vi "Handle Menu Selection.vi"(6 "Coords":T1, 8 "error in (no error)":errorcluster, 9 "Item Tag":string, 10 "Tree Refnum":refnum<vi>, 11 "Test Executive View in":refnum<class "Test Executive View.lvclass">) -> (0 "error out":errorcluster, 3 "Test Executive View out":refnum<class "Test Executive View.lvclass">)   [LabVIEW 2017, in "Test Executive View.lvclass"]
uses:
  Test Executive View.lvclass
  D:/Test-executive-builder/Source/Test Executive Builder View/Test Executive Builder View/Test Executive Builder View.lvclass
  <vilib>/Utility/miscctls.llb/LVPoint32TypeDef.ctl
  Source/Test Executive Builder View/Test Executive Builder View/Test Executive Builder View.lvclass/Test Executive Builder View.ctl
  Source/Application Dependencies/Insert While Loop.ctl
  Source/Application Dependencies/Insert For Loop.ctl
  Source/Application Dependencies/Insert Stop Loop.ctl
  Source/Application Dependencies/Insert Halt.ctl
  Source/Application Dependencies/Insert Test Step.ctl
  Source/Application Dependencies/Insert Subroutine.ctl
  Source/Application Dependencies/Insert Subsequence.ctl
  Source/Application Dependencies/Insert Conditional.ctl
  Source/Application Dependencies/Insert Case Structure.ctl
  Source/Application Dependencies/Insert Parallel.ctl
  Source/Test Executive Builder View/Tree Click Interpreter/Tree Click Interpreter.lvclass
  Source/Test Executive Builder View/Test Executive Builder View/Test Executive Builder View.lvclass
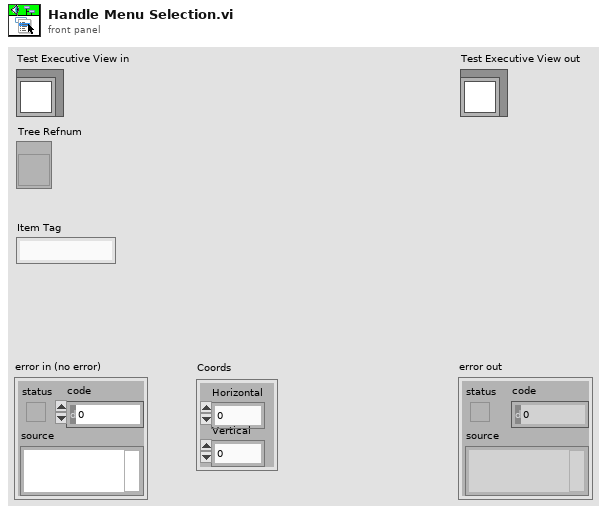
[diagram p1: front panel]
types:
  T1 = typedef "LVPoint32TypeDef.ctl" = cluster{"Horizontal":i32, "Vertical":i32}
  T2 = typedef "Insert While Loop.ctl" = cluster{"Parent ID":string, "Insertion Index":i32}
  T3 = typedef "Insert For Loop.ctl" = cluster{"Parent ID":string, "Insertion Index":i32, "Iterations":i32}
  T4 = typedef "Insert Stop Loop.ctl" = cluster{"Parent ID":string, "Insertion Index":i32}
  T5 = typedef "Insert Halt.ctl" = cluster{"Parent ID":string, "Insertion Index":i32}
  T6 = typedef "Insert Test Step.ctl" = cluster{"Parent ID":string, "Insertion Index":i32, "Test Step":string}
  T7 = typedef "Insert Subroutine.ctl" = cluster{"Parent ID":string, "Insertion Index":i32, "Path":path}
  T8 = typedef "Insert Subsequence.ctl" = cluster{"Parent ID":string, "Insertion Index":i32}
  T9 = typedef "Insert Conditional.ctl" = cluster{"Parent ID":string, "Insertion Index":i32}
  T10 = typedef "Insert Case Structure.ctl" = cluster{"Parent ID":string, "Insertion Index":i32}
  T11 = typedef "Insert Parallel.ctl" = cluster{"Parent ID":string, "Insertion Index":i32}
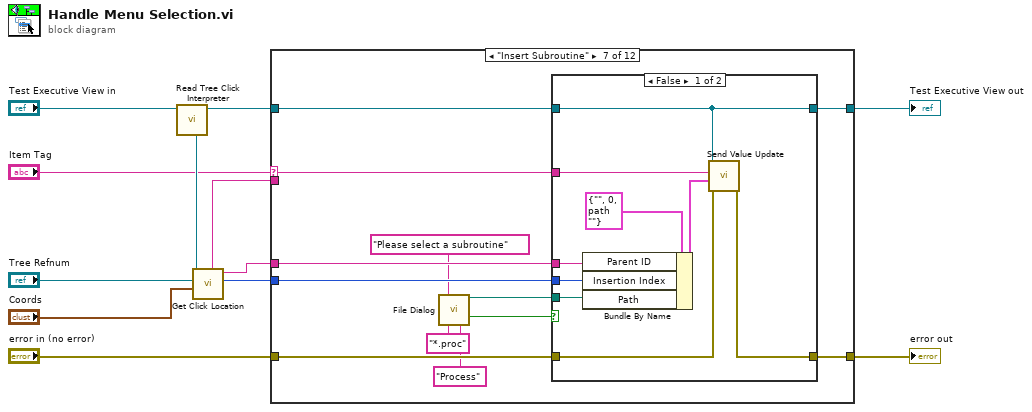
[diagram p0: block diagram]
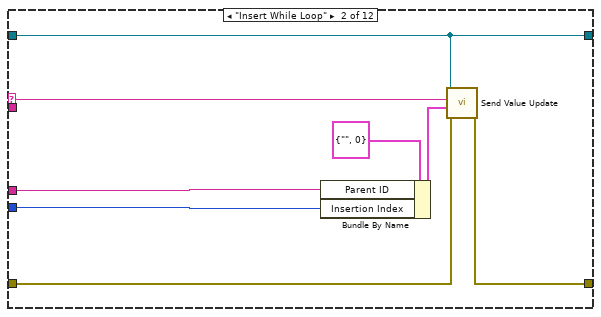
[diagram p3: hidden frame]
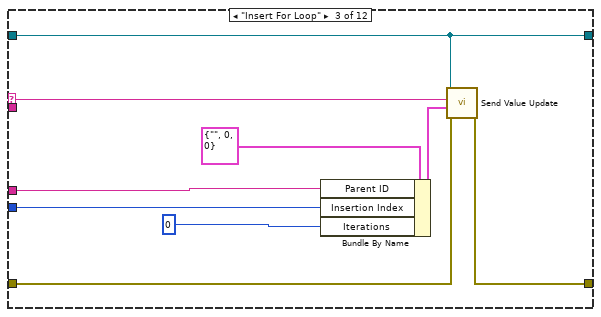
[diagram p4: hidden frame]
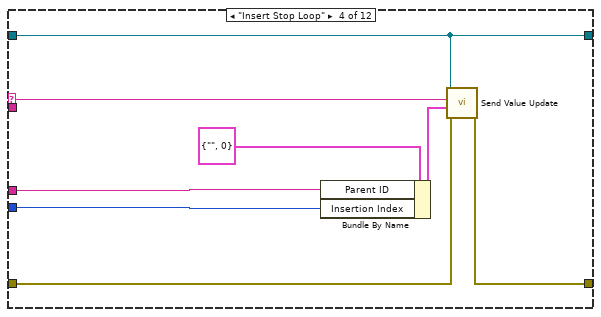
[diagram p5: hidden frame]
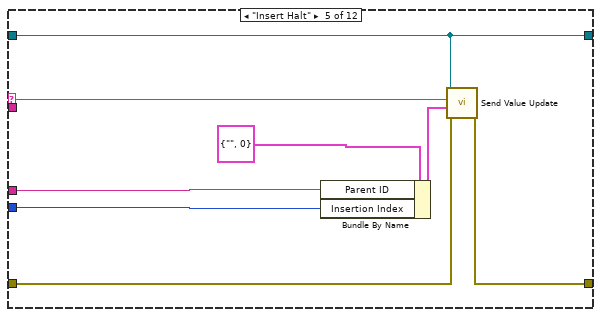
[diagram p6: hidden frame]
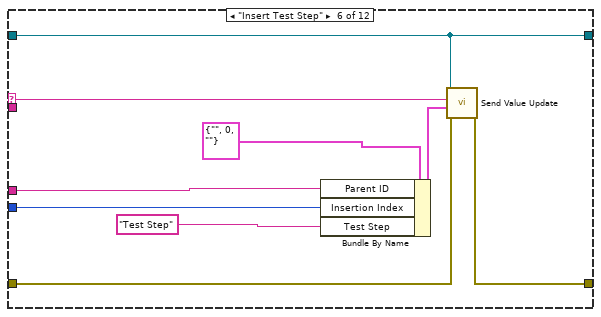
[diagram p7: hidden frame]
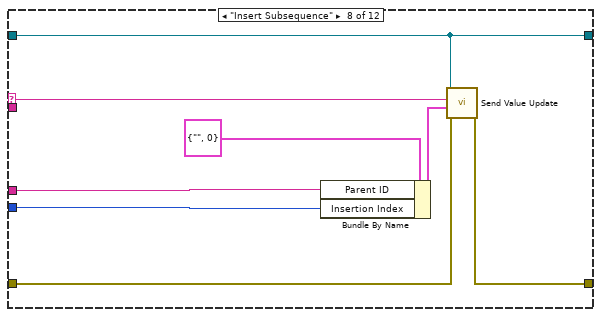
[diagram p9: hidden frame]
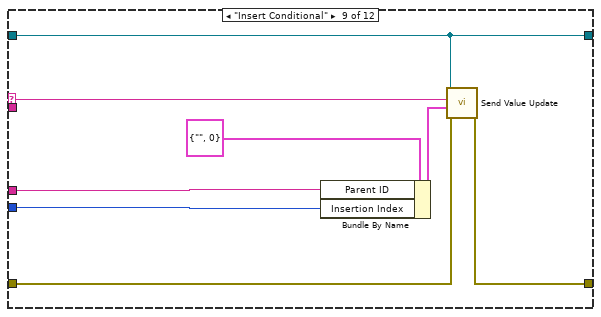
[diagram p10: hidden frame]
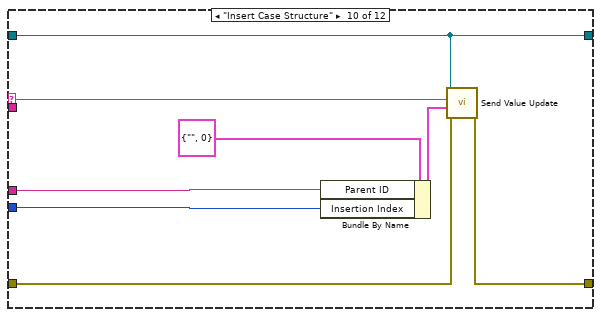
[diagram p11: hidden frame]
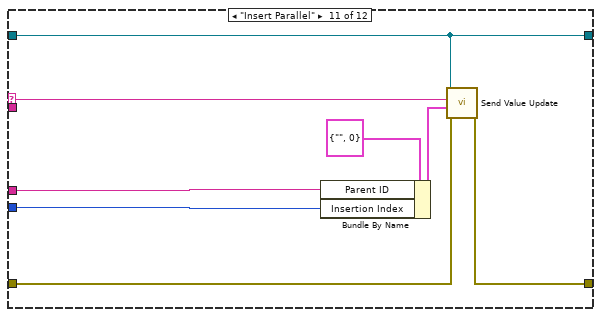
[diagram p12: hidden frame]
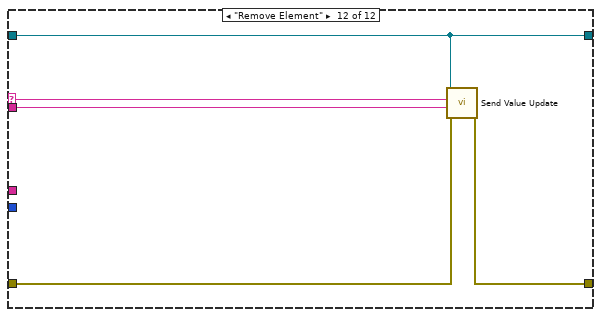
[diagram p13: hidden frame]
diagram:
  n1 = call "Read Tree Click Interpreter.vi"("Test Executive Builder View in"="Test Executive View in") -> ("Test Executive Builder View out"=w8:refnum<class "Test Executive View.lvclass">, "Tree Click Interpreter"=w7:refnum<class "Tree Click Interpreter.lvclass">)  [unwired: 9 in]
  n2 = call-dynamic "Get Click Location.vi"("Coords"="Coords", "Tree Refnum"="Tree Refnum", "Tree Click Interpreter in"=w7) -> ("Insertion Index"=w4:i32, "Parent ID"=w3:string, "Tag"=w1:string)  [unwired: 4 in, 2 out]
  n3 = case shown="\"Insert Subroutine\"" "Item Tag" {
    selector: "Item Tag" -> [_ w19 w28 w36 w44 w53 w65 w84 w92 w100 w108 w113]
    tunnel: [w14 w22 w31 w39 w47 w56 w60 w87 w95 w103 w111 w116] -> w12
    tunnel: w8 -> [w14 w22 w31 w39 w47 w56 w68 w87 w95 w103 w111 w116]
    tunnel: [w13 w20 w29 w37 w45 w54 w66 w85 w93 w101 w109 w114] -> w10
    tunnel: "error in (no error)" -> [w13 w21 w30 w38 w46 w55 w67 w86 w94 w102 w110 w115]
    tunnel: w4 -> [_ w18 w27 w35 w43 w52 w64 w83 w91 w99 w107 _]
    tunnel: w3 -> [_ w17 w26 w34 w42 w51 w63 w82 w90 w98 w106 _]
    tunnel: w1 -> [_ _ _ _ _ _ _ _ _ _ _ w112]
    frame Default {
    }
    frame "Insert While Loop" {
      n4 = Bundle By Name(cluster=T2 {"Parent ID"="", "Insertion Index"=0} ("Insert While Loop"), "Parent ID"=w17, "Insertion Index"=w18) -> (w15:T2)
      n5 = call-dynamic "Send Value Update.vi"("error in (no error)"=w21, "Value"=w15, "Datum Name"=w19, "IViewable in"=w22) -> ("error out"=w20:errorcluster)  [unwired: 7 in]
    }
    frame "Insert For Loop" {
      n6 = Bundle By Name(cluster=T3 {"Parent ID"="", "Insertion Index"=0, "Iterations"=0} ("Insert For Loop"), "Parent ID"=w26, "Insertion Index"=w27, "Iterations"=0) -> (w25:T3)
      n7 = call-dynamic "Send Value Update.vi"("error in (no error)"=w30, "Value"=w25, "Datum Name"=w28, "IViewable in"=w31) -> ("error out"=w29:errorcluster)  [unwired: 7 in]
    }
    frame "Insert Stop Loop" {
      n8 = Bundle By Name(cluster=T4 {"Parent ID"="", "Insertion Index"=0} ("Insert Stop Loop"), "Parent ID"=w34, "Insertion Index"=w35) -> (w33:T4)
      n9 = call-dynamic "Send Value Update.vi"("error in (no error)"=w38, "Value"=w33, "Datum Name"=w36, "IViewable in"=w39) -> ("error out"=w37:errorcluster)  [unwired: 7 in]
    }
    frame "Insert Halt" {
      n10 = Bundle By Name(cluster=T5 {"Parent ID"="", "Insertion Index"=0} ("Insert Halt"), "Parent ID"=w42, "Insertion Index"=w43) -> (w41:T5)
      n11 = call-dynamic "Send Value Update.vi"("error in (no error)"=w46, "Value"=w41, "Datum Name"=w44, "IViewable in"=w47) -> ("error out"=w45:errorcluster)  [unwired: 7 in]
    }
    frame "Insert Test Step" {
      n12 = Bundle By Name(cluster=T6 {"Parent ID"="", "Insertion Index"=0, "Test Step"=""} ("Insert Test Step"), "Parent ID"=w51, "Insertion Index"=w52, "Test Step"="Test Step") -> (w50:T6)
      n13 = call-dynamic "Send Value Update.vi"("error in (no error)"=w55, "Value"=w50, "Datum Name"=w53, "IViewable in"=w56) -> ("error out"=w54:errorcluster)  [unwired: 7 in]
    }
    frame "Insert Subroutine" {
      n14 = call "File Dialog"("prompt"="Please select a subroutine", "pattern (all files)"="*.proc", "pattern label"="Process") -> ("selected path"=w62:path, "cancelled"=w59:bool)  [unwired: 9 in, 2 out]
      n15 = case shown="False" w59 {
        tunnel: w68 -> [w69 w79]
        tunnel: w67 -> [w77 w78]
        tunnel: [w76 w78] -> w66
        tunnel: w65 -> [w75 _]
        tunnel: w64 -> [w74 _]
        tunnel: w63 -> [w73 _]
        tunnel: w62 -> [w70 _]
        tunnel: [w69 w79] -> w60
        frame False {
          n16 = Bundle By Name(cluster=T7 {"Parent ID"="", "Insertion Index"=0, "Path"=path ""} ("Insert Subroutine"), "Parent ID"=w73, "Insertion Index"=w74, "Path"=w70) -> (w72:T7)
          n17 = call-dynamic "Send Value Update.vi"("error in (no error)"=w77, "Value"=w72, "Datum Name"=w75, "IViewable in"=w69) -> ("error out"=w76:errorcluster)  [unwired: 7 in]
        }
        frame True {
        }
      }
    }
    frame "Insert Subsequence" {
      n18 = Bundle By Name(cluster=T8 {"Parent ID"="", "Insertion Index"=0} ("Insert Subsequence"), "Parent ID"=w82, "Insertion Index"=w83) -> (w81:T8)
      n19 = call-dynamic "Send Value Update.vi"("error in (no error)"=w86, "Value"=w81, "Datum Name"=w84, "IViewable in"=w87) -> ("error out"=w85:errorcluster)  [unwired: 7 in]
    }
    frame "Insert Conditional" {
      n20 = Bundle By Name(cluster=T9 {"Parent ID"="", "Insertion Index"=0} ("Insert Conditional"), "Parent ID"=w90, "Insertion Index"=w91) -> (w89:T9)
      n21 = call-dynamic "Send Value Update.vi"("error in (no error)"=w94, "Value"=w89, "Datum Name"=w92, "IViewable in"=w95) -> ("error out"=w93:errorcluster)  [unwired: 7 in]
    }
    frame "Insert Case Structure" {
      n22 = Bundle By Name(cluster=T10 {"Parent ID"="", "Insertion Index"=0} ("Insert Case Structure"), "Parent ID"=w98, "Insertion Index"=w99) -> (w97:T10)
      n23 = call-dynamic "Send Value Update.vi"("error in (no error)"=w102, "Value"=w97, "Datum Name"=w100, "IViewable in"=w103) -> ("error out"=w101:errorcluster)  [unwired: 7 in]
    }
    frame "Insert Parallel" {
      n24 = Bundle By Name(cluster=T11 {"Parent ID"="", "Insertion Index"=0} ("Insert Parallel"), "Parent ID"=w106, "Insertion Index"=w107) -> (w105:T11)
      n25 = call-dynamic "Send Value Update.vi"("error in (no error)"=w110, "Value"=w105, "Datum Name"=w108, "IViewable in"=w111) -> ("error out"=w109:errorcluster)  [unwired: 7 in]
    }
    frame "Remove Element" {
      n26 = call-dynamic "Send Value Update.vi"("error in (no error)"=w115, "Value"=w112, "Datum Name"=w113, "IViewable in"=w116) -> ("error out"=w114:errorcluster)  [unwired: 7 in]
    }
  }
  "error out" <- w10
  "Test Executive View out" <- w12
